vi "Inst.FP.GetPublicEvents.vi"(8 "error in (no error)":errorcluster, 11 "Inst.FP in":refnum<class "Inst.FP.lvclass">) -> (0 "error out":errorcluster, 2 "Inst.FP Public Events":T1, 3 "Inst.FP out":refnum<class "Inst.FP.lvclass">)   [LabVIEW 2019, in "Inst.FP.lvclass"]
uses:
  Inst.FP.lvclass
  <userlib>/LevyLab/RemoteControl/RemoteControl/Typedefs/Message--Cluster.ctl
  <userlib>/LevyLab/RemoteControl/RemoteControl/RemoteControl.lvclass
  Typedefs/PublicEvents--Inst.FP.MessageFromProcess.ctl
  Typedefs/PublicEvents--Cluster.ctl
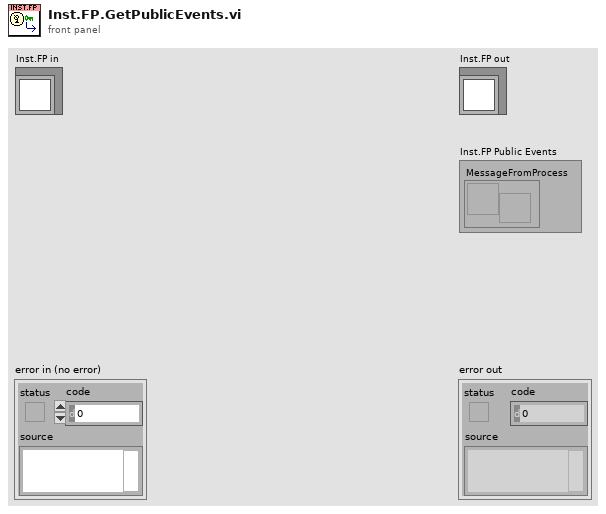
[diagram p1: front panel]
types:
  T1 = typedef "Inst.FP.lvclass/PublicEvents--Cluster.ctl" = cluster{"MessageFromProcess":refnum<user-event>}
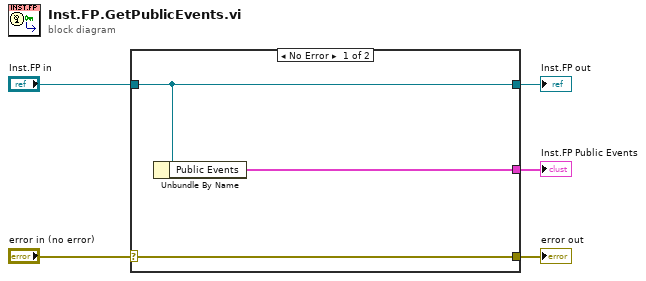
[diagram p0: block diagram]
diagram:
  n1 = case shown="No Error" "error in (no error)" {
    selector: "error in (no error)" -> [w8 w9]
    tunnel: [w8 w9] -> w4
    tunnel: [w7 w10] -> w2
    tunnel: "Inst.FP in" -> [w7 w10]
    tunnel: [w6 _] -> w1
    frame No Error {
      n2 = Unbundle By Name(w7) -> ("Public Events"=w6:T1)
    }
    frame Error {
    }
  }
  "error out" <- w4
  "Inst.FP out" <- w2
  "Inst.FP Public Events" <- w1
